vi "testFrequencyShift.vi"() -> ()   [LabVIEW 2012]
uses:
  <vilib>/Waveform/WDTOps.llb/WDT Get Waveform Time Array DBL.vi
  <vilib>/Analysis/2dsp.llb/Real FFT.vi
  <vilib>/Analysis/2dsp.llb/Inverse Real FFT.vi
  <vilib>/Analysis/NI_AALPro.lvlib
panel:
  out "Waveform Graph 4":waveform(dbl)(graph)
  out "Waveform Graph 3":dbl[](graph)
  out "Waveform Graph 2":waveform(dbl)(graph)
  out "Waveform Graph":dynamicdata(graph)
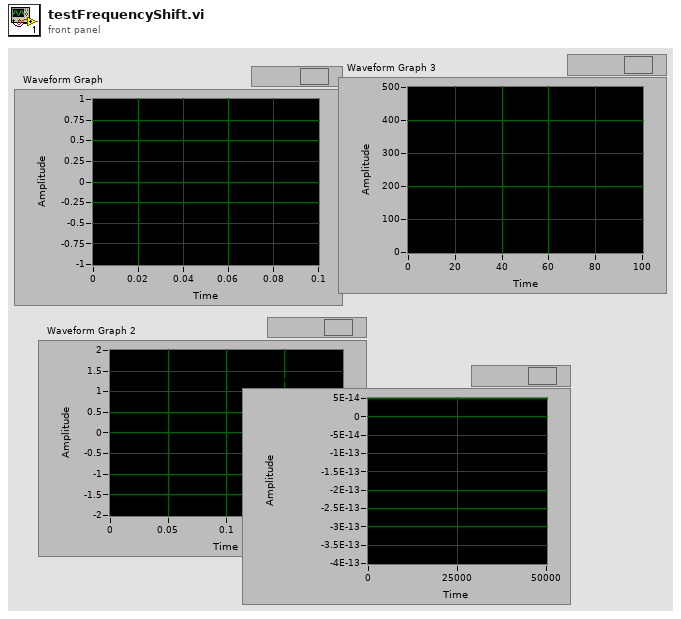
[diagram p1: front panel]
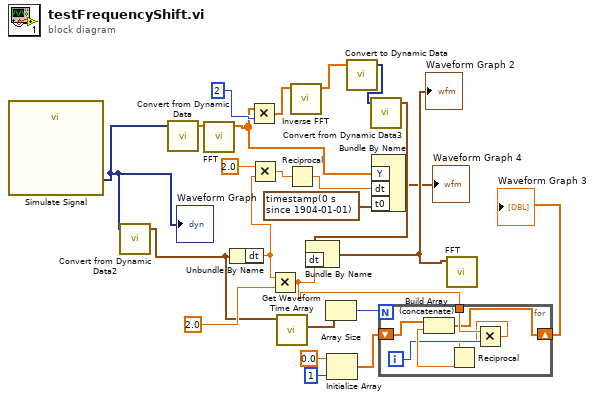
[diagram p0: block diagram]
diagram:
  n1 = call "Simulate Signal"() -> ("Sine"=w23:dynamicdata)  [unwired: 14 in, 1 out]
  "Waveform Graph" <- w23
  n2 = call "Convert from Dynamic Data2"("Dynamic Data Type"=w23) -> ("Waveform"=w15:waveform(dbl))  [unwired: 3 in]
  n3 = call "Convert from Dynamic Data"("Dynamic Data Type"=w23) -> ("Array"=w24:dbl[])  [unwired: 3 in]
  n4 = call-poly <vilib>:"FFT.vi"("X"=w24) -> ("FFT {X}"=w1:cdb[])  [unwired: 9 in, 1 out]
  n5 = Unbundle By Name(w15) -> ("dt"=w7:dbl)
  n6 = Multiply(x=w1, y=2) -> (x*y=w9:cdb[])
  n7 = Multiply(x=2.0, y=w7) -> (x*y=w5:dbl)
  n8 = Multiply(x=w7, y=2.0) -> (x*y=w10:dbl)
  n9 = call-poly <vilib>:"Get Waveform Time Array.vi"("waveform in"=w15) -> ("X array"=w16:timestamp[])  [unwired: 9 in, 1 out]
  n10 = Reciprocal(x=w5) -> (1/x=w3:dbl)
  n11 = call-poly <vilib>:"Inverse FFT.vi"("FFT {X}"=w9) -> ("X"=w22:dbl[])  [unwired: 9 in, 1 out]
  n12 = Array Size(array=w16) -> (size(s)=w14:i32)
  n13 = Initialize Array(0.0 ("element"), 1 ("dimension size")) -> (w13:dbl[])
  n14 = call "Convert to Dynamic Data"("Array"=w22) -> ("Dynamic Data Type"=w21:dynamicdata)  [unwired: 3 in]
  n15 = call "Convert from Dynamic Data3"("Dynamic Data Type"=w21) -> ("Waveform"=w20:waveform(dbl))  [unwired: 3 in]
  n16 = Bundle By Name(cluster=w20, "dt"=w10) -> (w17:waveform(dbl))
  "Waveform Graph 2" <- w17
  n17 = Bundle By Name("Y"=w1, "dt"=w3, "t0"=timestamp(0 s since 1904-01-01)) -> (→"Waveform Graph 4":waveform(cdb))  [unwired: 1 in]
  n18 = for {
    N: w14 -> [_]
    shift-right: [w25] -> w8
    shift-left: w13 -> [w30]
    tunnel: w10 -> [w28]
    i -> [w27]
    n19 = Multiply(x=w28, y=w27) -> (x*y=w26:dbl)
    n20 = Reciprocal(x=w26) -> (1/x=w29:dbl)
    n21 = Build Array (concatenate)(w30, w29) -> (w25:dbl[])
  }
  "Waveform Graph 3" <- w8
  n22 = call-poly <vilib>:"FFT.vi"("X"=w17) -> ()  [unwired: 9 in, 2 out]
